vi "Color Editor.vi"(9 "Min":sgl, 10 "Max":sgl=10.0, 11 "Color Ramp Cluster in":T1={"Color Ramp Style"=enum."None", "Color Ramp Array"=[16711934, 393471, 57855, 4390754, 16449346, 16744722, 16711680], "Color Ramp Index"=[45, 91, 133, 175, 219, 255], "Interpolate?"=FALSE, "Logarithm?"=FALSE}) -> (3 "Color Ramp Cluster out":T1={"Color Ramp Style"=enum."None", "Color Ramp Array"=[16711934, 393471, 57855, 4390754, 16449346, 16744722, 16711680], "Color Ramp Index"=[45, 91, 133, 175, 219, 255], "Interpolate?"=FALSE, "Logarithm?"=FALSE})   [LabVIEW 2020, in "3D Plot.lvclass"]
uses:
  <vilib>/Math Plots/3D Math Plots/3D Plot/3D Plot/3D Plot.lvclass
  <vilib>/Math Plots/3D Math Plots/3D Plot/3D Plot/Typedef/Color Ramp Cluster.ctl
  <vilib>/Math Plots/3D Math Plots/3D Plot/3D Plot/Typedef/Color Editor State.ctl
panel:
  in  "Tab Control":enum32{"UI", "Input & Output"}(tab)
  in  "Help":bool
  out "Intensity Graph":dbl[][](graph)
  in  "Slider 10":i32(slide) scale=0.0..255.0
  in  "Numeric 10":sgl=50.0
  in  "Color 10":u32(colorbox)=6618880
  in  "Slider 9":i32(slide) scale=0.0..255.0
  in  "Numeric 9":sgl=50.0
  in  "Color 9":u32(colorbox)=6618880
  in  "Slider 8":i32(slide) scale=0.0..255.0
  in  "Numeric 8":sgl=50.0
  in  "Color 8":u32(colorbox)=6618880
  in  "Slider 7":i32(slide) scale=0.0..255.0
  in  "Numeric 7":sgl=50.0
  in  "Color 7":u32(colorbox)=6618880
  in  "Slider 6":i32(slide) scale=0.0..255.0
  in  "Numeric 6":sgl=50.0
  in  "Color 6":u32(colorbox)=6618880
  in  "Slider 5":i32(slide) scale=0.0..255.0
  in  "Numeric 5":sgl=50.0
  in  "Color 5":u32(colorbox)=6618880
  in  "Slider 4":i32(slide) scale=0.0..255.0
  in  "Numeric 4":sgl=50.0
  in  "Color 4":u32(colorbox)=6618880
  in  "Slider 3":i32(slide) scale=0.0..255.0
  in  "Numeric 3":sgl=50.0
  in  "Color 3":u32(colorbox)=6618880
  in  "Slider 2":i32(slide) scale=0.0..255.0
  in  "Numeric 2":sgl=50.0
  in  "Color 2":u32(colorbox)=6618880
  in  "Slider 1":i32(slide) scale=0.0..255.0
  in  "Numeric 1":sgl=50.0
  in  "Color 1":u32(colorbox)=6618880
  in  "Logarithm":bool
  in  "Interpolate":bool
  in  "Bottom Numeric":sgl
  in  "Top Numeric":sgl=100.0
  in  "Bottom Color":u32(colorbox)=16860
  in  "Top Color":u32(colorbox)=16711680
  in  "Delete":bool
  in  "Add":bool
  in  "Cancel":bool
  in  "OK":bool
  in  "Bounds Slider":cluster{u8, u8}(slide)={0, 255} scale=0.0..255.0
  in  "Active Slider ID":i32
  # "Color Ramp"
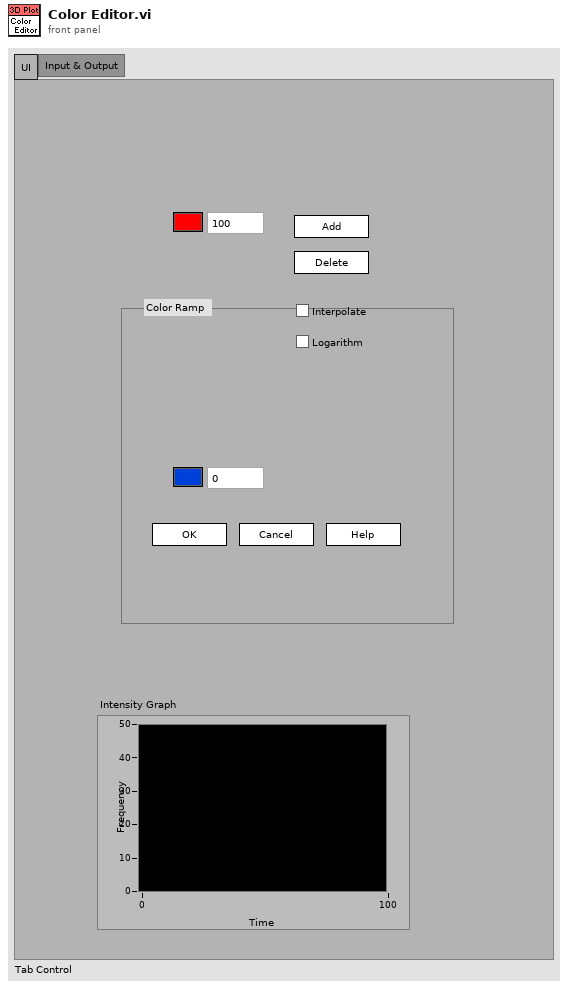
[diagram p1: front panel]
types:
  T1 = typedef "3D Plot.lvclass/Color Ramp Cluster.ctl" = cluster{"Color Ramp Style":enum16{"None", "Shaded", "Color spectrum", "Grey scale", "Custom"}, "Color Ramp Array":u32[], "Color Ramp Index":i32[], "Interpolate?":bool, "Logarithm?":bool}
  T2 = enum16{"None", "Shaded", "Color spectrum", "Grey scale", "Custom"}
  T3 = typedef "3D Plot.lvclass/Color Editor State.ctl" = enum16{"OK Pressed", "Cancel Pressed", "Update Color Ramp", "Update Height bySlider", "Update Height by Numeric", "Logarithm Color Ramp", "Set Active Slider", "Add a New Item", "Delete the Item"}
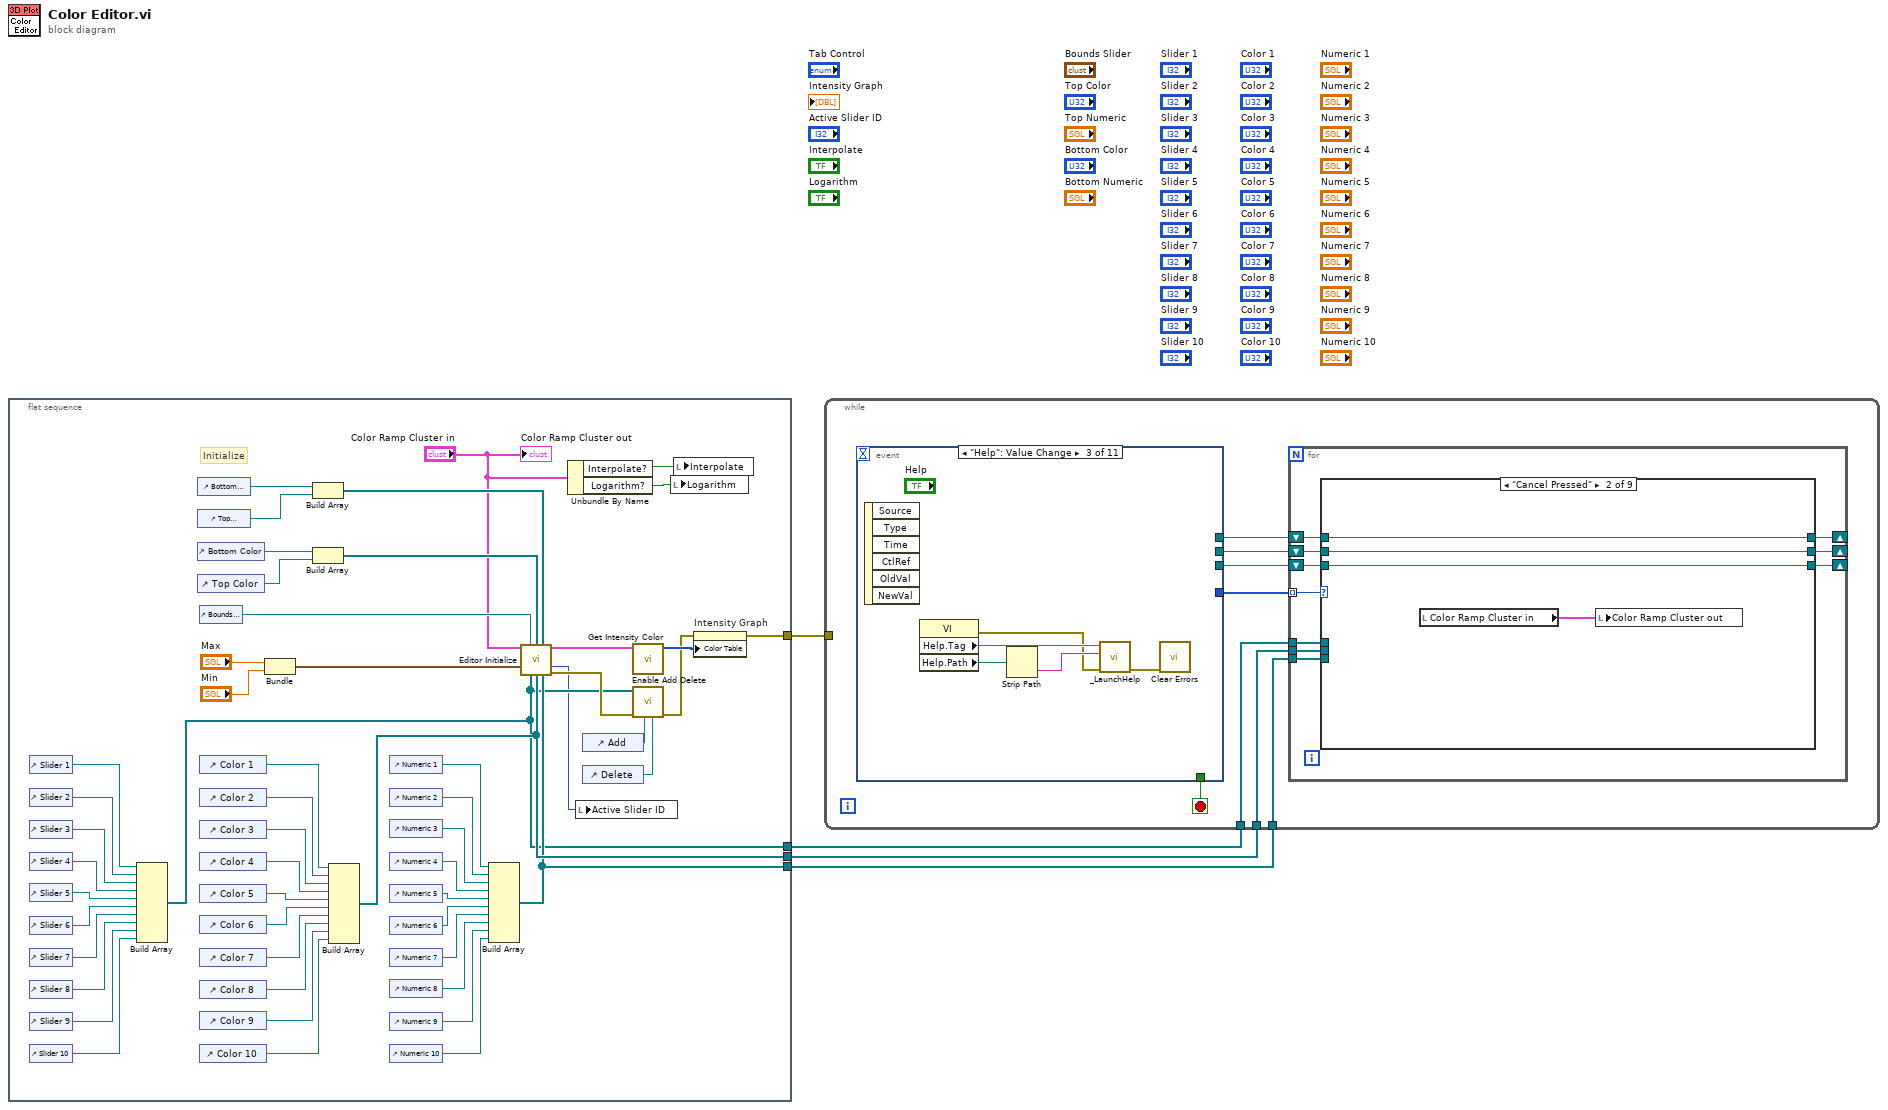
[diagram p0: block diagram]
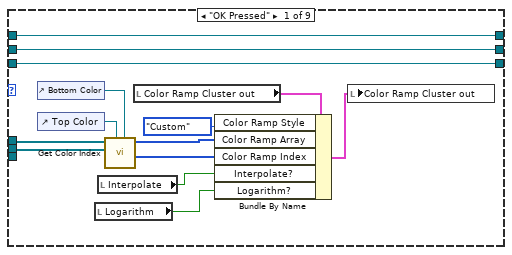
[diagram p2: hidden frame]
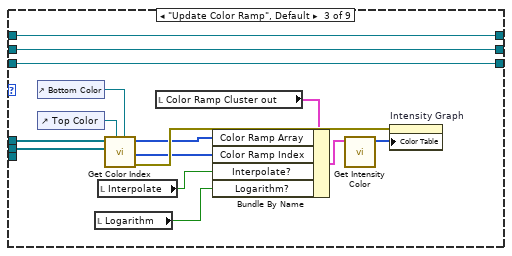
[diagram p3: hidden frame]
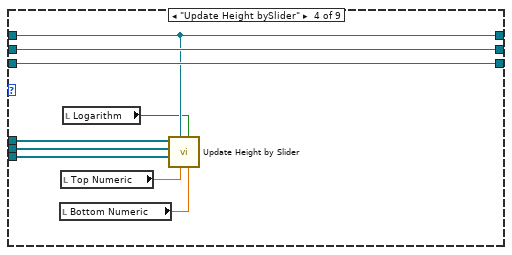
[diagram p4: hidden frame]
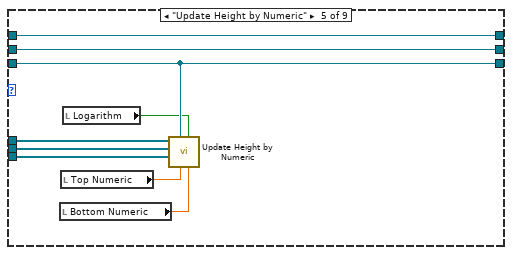
[diagram p5: hidden frame]
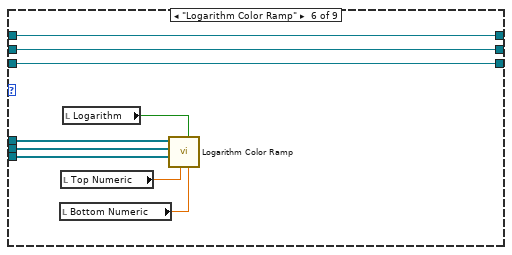
[diagram p6: hidden frame]
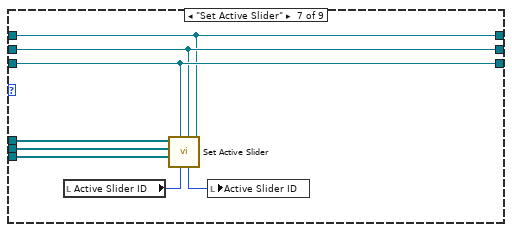
[diagram p7: hidden frame]
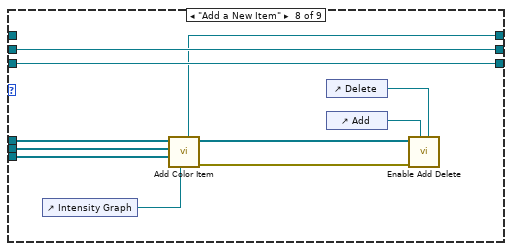
[diagram p8: hidden frame]
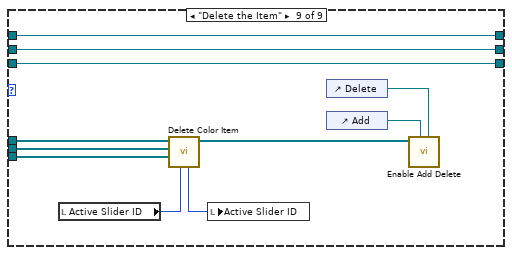
[diagram p9: hidden frame]
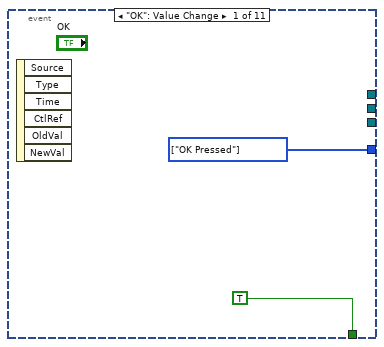
[diagram p10: hidden frame]
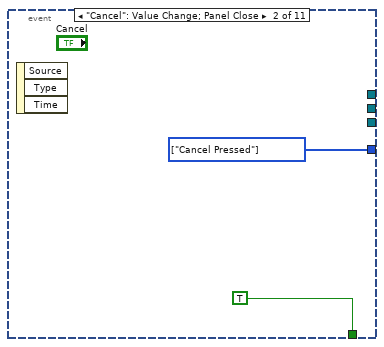
[diagram p11: hidden frame]
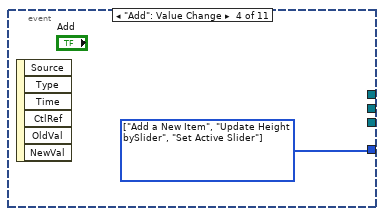
[diagram p12: hidden frame]
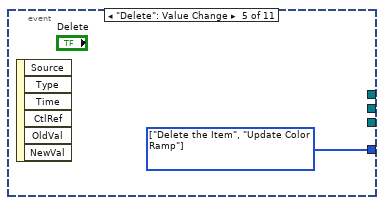
[diagram p13: hidden frame]
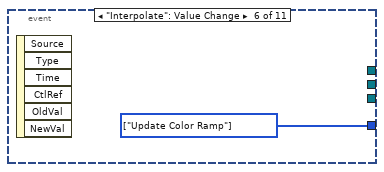
[diagram p14: hidden frame]
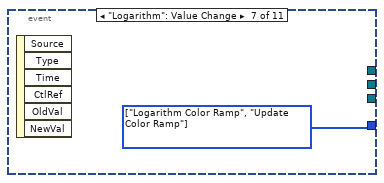
[diagram p15: hidden frame]
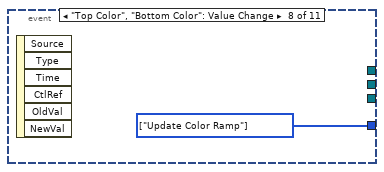
[diagram p16: hidden frame]
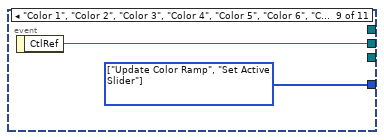
[diagram p17: hidden frame]
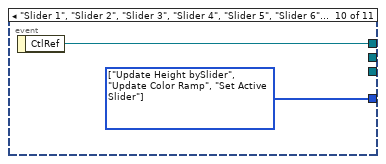
[diagram p18: hidden frame]
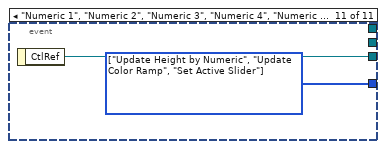
[diagram p19: hidden frame]
diagram:
  n1 = flat-sequence {
    tunnel: [w57] -> w4
    tunnel: [w10] -> w3
    tunnel: [w12] -> w2
    tunnel: [w11] -> w1
    frame #0 {
      # "Initialize"
      n2 = control-ref of="Slider 1"() -> (w21:refnum<vi>)
      n3 = control-ref of="Slider 2"() -> (w28:refnum<vi>)
      n4 = control-ref of="Slider 3"() -> (w29:refnum<vi>)
      n5 = control-ref of="Slider 4"() -> (w30:refnum<vi>)
      n6 = control-ref of="Slider 5"() -> (w31:refnum<vi>)
      n7 = control-ref of="Slider 6"() -> (w32:refnum<vi>)
      n8 = control-ref of="Slider 7"() -> (w33:refnum<vi>)
      n9 = control-ref of="Slider 8"() -> (w34:refnum<vi>)
      n10 = control-ref of="Slider 9"() -> (w35:refnum<vi>)
      n11 = control-ref of="Slider 10"() -> (w36:refnum<vi>)
      n12 = Build Array(w21, w28, w29, w30, w31, w32, w33, w34, w35, w36) -> (w10:refnum<vi>[])
      n13 = control-ref of="Bottom Numeric"() -> (w25:refnum<vi>)
      n14 = control-ref of="Top Numeric"() -> (w24:refnum<vi>)
      n15 = control-ref of="Bottom Color"() -> (w27:refnum<vi>)
      n16 = control-ref of="Top Color"() -> (w26:refnum<vi>)
      n17 = control-ref of="Bounds Slider"() -> (w20:refnum<vi>)
      n18 = control-ref of="Color 1"() -> (w47:refnum<vi>)
      n19 = control-ref of="Color 2"() -> (w48:refnum<vi>)
      n20 = control-ref of="Color 3"() -> (w49:refnum<vi>)
      n21 = control-ref of="Color 4"() -> (w50:refnum<vi>)
      n22 = control-ref of="Color 5"() -> (w51:refnum<vi>)
      n23 = control-ref of="Color 6"() -> (w52:refnum<vi>)
      n24 = control-ref of="Color 7"() -> (w53:refnum<vi>)
      n25 = control-ref of="Color 8"() -> (w54:refnum<vi>)
      n26 = control-ref of="Color 9"() -> (w55:refnum<vi>)
      n27 = control-ref of="Color 10"() -> (w56:refnum<vi>)
      n28 = Bundle("Max"="Max", "Min"="Min") -> (w15:cluster{"Max":sgl, "Min":sgl})  [unwired: 1 out]
      n29 = Build Array(w25, w24) -> (w22:refnum<vi>[])
      n30 = Build Array(w27, w26) -> (w23:refnum<vi>[])
      n31 = Build Array(w47, w48, w49, w50, w51, w52, w53, w54, w55, w56) -> (w12:refnum<vi>[])
      n32 = control-ref of="Numeric 1"() -> (w37:refnum<vi>)
      n33 = control-ref of="Numeric 2"() -> (w38:refnum<vi>)
      n34 = control-ref of="Numeric 3"() -> (w39:refnum<vi>)
      n35 = control-ref of="Numeric 4"() -> (w40:refnum<vi>)
      n36 = control-ref of="Numeric 5"() -> (w41:refnum<vi>)
      n37 = control-ref of="Numeric 6"() -> (w42:refnum<vi>)
      n38 = control-ref of="Numeric 7"() -> (w43:refnum<vi>)
      n39 = control-ref of="Numeric 8"() -> (w44:refnum<vi>)
      n40 = control-ref of="Numeric 9"() -> (w45:refnum<vi>)
      n41 = control-ref of="Numeric 10"() -> (w46:refnum<vi>)
      n42 = Build Array(w37, w38, w39, w40, w41, w42, w43, w44, w45, w46) -> (w11:refnum<vi>[])
      n43 = call <vilib>:"Editor Initialize.vi"("Color Ramp Cluster in"="Color Ramp Cluster in", "Fixed Slider Ref"=w20, "Fixed Color Ref Array"=w23, "Fixed Numeric Ref Array"=w22, "Range In"=w15, "Slider Ref Array"=w10, "Color Ref Array"=w12, "Numeric Ref Array"=w11) -> ("Color Ramp Cluster out"=w8:T1, "Active Slider ID"=w9:i32, "error out"=w14:errorcluster)  [unwired: 4 in, 1 out]
      n44 = Unbundle By Name("Color Ramp Cluster in") -> ("Interpolate?"=w7:bool, "Logarithm?"=w6:bool)
      n45 = local write "Active Slider ID"(w9) -> ()
      n46 = control-ref of="Add"() -> (w19:refnum<vi>)
      n47 = control-ref of="Delete"() -> (w18:refnum<vi>)
      n48 = call <vilib>:"Get Intensity Color.vi"("Color Ramp Cluster"=w8) -> ("Intensity Color"=w58:u32[])  [unwired: 4 in, 6 out]
      n49 = call <vilib>:"Enable Add Delete.vi"("Delete Ref"=w18, "Add Ref"=w19, "error in (no error)"=w14, "Slider Ref Array"=w10) -> ("error out"=w13:errorcluster)  [unwired: 7 out]
      n50 = local write "Logarithm"(w6) -> ()
      n51 = local write "Interpolate"(w7) -> ()
      n52 = property on="Intensity Graph" class="IntGraph (strict)"(error in=w13, "Color Table"=w58) -> (error out=w57:errorcluster)  [unwired: 1 in, 1 out]
      "Color Ramp Cluster out" <- "Color Ramp Cluster in"
    }
  }
  n53 = while {
    tunnel: w4 -> [_]
    tunnel: w1 -> [w62]
    tunnel: w2 -> [w65]
    tunnel: w3 -> [w63]
    stop <- w66 stop-if-true
    n54 = event shown="[2] \"Help\": Value Change" {
      selector: _ -> [_ _ _ _ _ _ _ _ _ _ _]
      dyn-events: _ -> [_ _ _ _ _ _ _ _ _ _ _]
      timeout: _ -> [_ _ _ _ _ _ _ _ _ _ _]
      tunnel: [TRUE TRUE ("OK") _ _ _ _ _ _ _ _ _] -> w66
      tunnel: [w166 w168 _ w174 w175 w176 w177 w178 w180 w181 w183] -> w64
      tunnel: [_ _ _ _ _ _ _ _ _ w182 _] -> w59
      tunnel: [_ _ _ _ _ _ _ _ _ _ w184] -> w60
      tunnel: [_ _ _ _ _ _ _ _ w179 _ _] -> w61
      event "OK": Value Change {
        w166 = T3[] [enum."OK Pressed"] items=["OK Pressed", "Cancel Pressed", "Update Color Ramp", "Update Height bySlider", "Update Height by Numeric", "Logarithm Color Ramp", "Set Active Slider", "Add a New Item", "Delete the Item"]
        n55 = event-data() -> ()  [unwired: 7 out]
      }
      event "Cancel": Value Change; Panel Close {
        w168 = T3[] [enum."Cancel Pressed"] items=["OK Pressed", "Cancel Pressed", "Update Color Ramp", "Update Height bySlider", "Update Height by Numeric", "Logarithm Color Ramp", "Set Active Slider", "Add a New Item", "Delete the Item"]
        n56 = event-data() -> ()  [unwired: 4 out]
      }
      event "Help": Value Change {
        n57 = event-data() -> ()  [unwired: 7 out]
        n58 = property class="VI"() -> (error out=w170:errorcluster, "Help.Tag"=w172:string, "Help.Path"=w173:path)  [unwired: 2 in, 1 out]
        n59 = Strip Path(path=w173) -> (name=w171:string)  [unwired: 1 out]
        n60 = call <helpdir>:"_LaunchHelp.vi"("error in (no error)"=w170, "CHM or HLP filename (lvdialog.chm)"=w171, "HTML filename"=w172) -> ("error out"=w169:errorcluster)  [unwired: 4 out]
        n61 = call <vilib>:"Clear Errors.vi"("error in (no error)"=w169) -> ()  [unwired: 5 in, 2 out]
      }
      event "Add": Value Change {
        w174 = T3[] [enum."Add a New Item", enum."Update Height bySlider", enum."Set Active Slider"] items=["OK Pressed", "Cancel Pressed", "Update Color Ramp", "Update Height bySlider", "Update Height by Numeric", "Logarithm Color Ramp", "Set Active Slider", "Add a New Item", "Delete the Item"]
        n62 = event-data() -> ()  [unwired: 7 out]
      }
      event "Delete": Value Change {
        w175 = T3[] [enum."Delete the Item", enum."Update Color Ramp"] items=["OK Pressed", "Cancel Pressed", "Update Color Ramp", "Update Height bySlider", "Update Height by Numeric", "Logarithm Color Ramp", "Set Active Slider", "Add a New Item", "Delete the Item"] ("Array")
        n63 = event-data() -> ()  [unwired: 7 out]
      }
      event "Interpolate": Value Change {
        w176 = T3[] [enum."Update Color Ramp"] items=["OK Pressed", "Cancel Pressed", "Update Color Ramp", "Update Height bySlider", "Update Height by Numeric", "Logarithm Color Ramp", "Set Active Slider", "Add a New Item", "Delete the Item"]
        n64 = event-data() -> ()  [unwired: 7 out]
      }
      event "Logarithm": Value Change {
        w177 = T3[] [enum."Logarithm Color Ramp", enum."Update Color Ramp"] items=["OK Pressed", "Cancel Pressed", "Update Color Ramp", "Update Height bySlider", "Update Height by Numeric", "Logarithm Color Ramp", "Set Active Slider", "Add a New Item", "Delete the Item"] ("Array")
        n65 = event-data() -> ()  [unwired: 7 out]
      }
      event "Top Color", "Bottom Color": Value Change {
        w178 = T3[] [enum."Update Color Ramp"] items=["OK Pressed", "Cancel Pressed", "Update Color Ramp", "Update Height bySlider", "Update Height by Numeric", "Logarithm Color Ramp", "Set Active Slider", "Add a New Item", "Delete the Item"]
        n66 = event-data() -> ()  [unwired: 7 out]
      }
      event "Color 1", "Color 2", "Color 3", "Color 4", "Color 5", "Color 6", "Color 7", "Color 8", "Color 9", "Color 10": Value Change {
        w180 = T3[] [enum."Update Color Ramp", enum."Set Active Slider"] items=["OK Pressed", "Cancel Pressed", "Update Color Ramp", "Update Height bySlider", "Update Height by Numeric", "Logarithm Color Ramp", "Set Active Slider", "Add a New Item", "Delete the Item"]
        n67 = event-data() -> ("CtlRef"=w179:refnum<vi>)  [unwired: 1 out]
      }
      event "Slider 1", "Slider 2", "Slider 3", "Slider 4", "Slider 5", "Slider 6", "Slider 7", "Slider 8", "Slider 9", "Slider 10": Value Change {
        w181 = T3[] [enum."Update Height bySlider", enum."Update Color Ramp", enum."Set Active Slider"] items=["OK Pressed", "Cancel Pressed", "Update Color Ramp", "Update Height bySlider", "Update Height by Numeric", "Logarithm Color Ramp", "Set Active Slider", "Add a New Item", "Delete the Item"]
        n68 = event-data() -> ("CtlRef"=w182:refnum<vi>)  [unwired: 1 out]
      }
      event "Numeric 1", "Numeric 2", "Numeric 3", "Numeric 4", "Numeric 5", "Numeric 6", "Numeric 7", "Numeric 8", "Numeric 9", "Numeric 10": Value Change {
        w183 = T3[] [enum."Update Height by Numeric", enum."Update Color Ramp", enum."Set Active Slider"] items=["OK Pressed", "Cancel Pressed", "Update Color Ramp", "Update Height bySlider", "Update Height by Numeric", "Logarithm Color Ramp", "Set Active Slider", "Add a New Item", "Delete the Item"]
        n69 = event-data() -> ("CtlRef"=w184:refnum<vi>)  [unwired: 1 out]
      }
    }
    n70 = for {
      tunnel: w63 -> [w76]
      tunnel: w65 -> [w75]
      tunnel: w64 -> [w74] mode=indexing
      tunnel: w62 -> [w73]
      shift-right: [w69] -> _
      shift-left: w59 -> [w70]
      shift-right: [w68] -> _
      shift-left: w61 -> [w72]
      shift-right: [w67] -> _
      shift-left: w60 -> [w71]
      n71 = case shown="\"Cancel Pressed\"" w74 {
        tunnel: w76 -> [w81 _ w107 w114 w125 w133 w144 w147 w157]
        tunnel: w75 -> [w80 _ w106 w116 w124 w132 w142 w153 w160]
        tunnel: w70 -> [w90 w93 w104 w111 w120 w136 w139 _ w164]
        tunnel: w73 -> [_ _ _ w115 w123 w131 w143 w152 w159]
        tunnel: w71 -> [w88 w91 w102 w112 w122 w134 w141 w150 w162]
        tunnel: w72 -> [w89 w92 w103 w113 w121 w135 w140 w151 w163]
        tunnel: [w90 w93 w104 w111 w120 w136 w139 w146 w164] -> w69
        tunnel: [w89 w92 w103 w113 w121 w135 w140 w151 w163] -> w68
        tunnel: [w88 w91 w102 w112 w122 w134 w141 w150 w162] -> w67
        frame "OK Pressed" {
          n72 = control-ref of="Bottom Color"() -> (w86:refnum<vi>)
          n73 = control-ref of="Top Color"() -> (w87:refnum<vi>)
          n74 = local read "Logarithm"() -> (w77:bool)
          n75 = local read "Interpolate"() -> (w78:bool)
          n76 = call <vilib>:"Get Color Index.vi"("Bottom Color Ref"=w86, "Top Color Ref"=w87, "Color Ref Array"=w80, "Slider Ref Array"=w81) -> ("Color Ramp Index"=w83:i32[], "Color Ramp Array"=w84:u32[])  [unwired: 1 in, 5 out]
          n77 = local read "Color Ramp Cluster out"() -> (w85:T1)
          n78 = Bundle By Name(cluster=w85, "Color Ramp Style"=T2."Custom", "Color Ramp Array"=w84, "Color Ramp Index"=w83, "Interpolate?"=w78, "Logarithm?"=w77) -> (w82:T1)
          n79 = local write "Color Ramp Cluster out"(w82) -> ()
        }
        frame "Cancel Pressed" {
          n80 = local read "Color Ramp Cluster in"() -> (w94:T1)
          n81 = local write "Color Ramp Cluster out"(w94) -> ()
        }
        frame "Update Color Ramp", Default {
          n82 = control-ref of="Bottom Color"() -> (w108:refnum<vi>)
          n83 = control-ref of="Top Color"() -> (w109:refnum<vi>)
          n84 = local read "Logarithm"() -> (w96:bool)
          n85 = local read "Interpolate"() -> (w97:bool)
          n86 = call <vilib>:"Get Color Index.vi"("Bottom Color Ref"=w108, "Top Color Ref"=w109, "Color Ref Array"=w106, "Slider Ref Array"=w107) -> ("error out"=w101:errorcluster, "Color Ramp Index"=w98:i32[], "Color Ramp Array"=w99:u32[])  [unwired: 1 in, 4 out]
          n87 = local read "Color Ramp Cluster out"() -> (w100:T1)
          n88 = Bundle By Name(cluster=w100, "Color Ramp Array"=w99, "Color Ramp Index"=w98, "Interpolate?"=w97, "Logarithm?"=w96) -> (w95:T1)
          n89 = call <vilib>:"Get Intensity Color.vi"("Color Ramp Cluster"=w95) -> ("Intensity Color"=w105:u32[])  [unwired: 4 in, 6 out]
          n90 = property on="Intensity Graph" class="IntGraph (strict)"(error in=w101, "Color Table"=w105) -> ()  [unwired: 1 in, 2 out]
        }
        frame "Update Height bySlider" {
          n91 = local read "Bottom Numeric"() -> (w118:sgl)
          n92 = local read "Top Numeric"() -> (w117:sgl)
          n93 = local read "Logarithm"() -> (w110:bool)
          n94 = call <vilib>:"Update Height by Slider.vi"("Bottom Numeric"=w118, "Logarithm?"=w110, "Top Numeric"=w117, "Slider Ref"=w111, "Numeric Ref Array"=w115, "Color Ref Array"=w116, "Slider Ref Array"=w114) -> ()  [unwired: 1 in, 4 out]
        }
        frame "Update Height by Numeric" {
          n95 = local read "Bottom Numeric"() -> (w127:sgl)
          n96 = local read "Top Numeric"() -> (w126:sgl)
          n97 = local read "Logarithm"() -> (w119:bool)
          n98 = call <vilib>:"Update Height by Numeric.vi"("Bottom Numeric"=w127, "Logarithm?"=w119, "Top Numeric"=w126, "Active Numeric Ref"=w122, "Numeric Ref Array"=w123, "Color Ref Array"=w124, "Slider Ref Array"=w125) -> ()  [unwired: 1 in, 4 out]
        }
        frame "Logarithm Color Ramp" {
          n99 = local read "Bottom Numeric"() -> (w128:sgl)
          n100 = local read "Top Numeric"() -> (w129:sgl)
          n101 = local read "Logarithm"() -> (w130:bool)
          n102 = call <vilib>:"Logarithm Color Ramp.vi"("Bottom Numeric"=w128, "Logarithm?"=w130, "Top Numeric"=w129, "Numeric Ref Array"=w131, "Color Ref Array"=w132, "Slider Ref Array"=w133) -> ()  [unwired: 1 in, 5 out]
        }
        frame "Set Active Slider" {
          n103 = local read "Active Slider ID"() -> (w138:i32)
          n104 = call <vilib>:"Set Active Slider.vi"("Slider Ref"=w139, "Color Ref"=w140, "Ex Active Slider ID"=w138, "Numeric Ref"=w141, "Numeric Ref Array"=w143, "Color Ref Array"=w142, "Slider Ref Array"=w144) -> ("New Active Slider ID"=w137:i32)  [unwired: 1 in, 3 out]
          n105 = local write "Active Slider ID"(w137) -> ()
        }
        frame "Add a New Item" {
          n106 = control-ref of="Intensity Graph"() -> (w154:refnum<vi>)
          n107 = call <vilib>:"Add Color Item.vi"("Color Ramp Ref"=w154, "Numeric Ref Array In"=w152, "Color Ref Array In"=w153, "Slider Ref Array"=w147) -> ("error out"=w145:errorcluster, "Slider Ref"=w146:refnum<vi>)  [unwired: 1 in, 5 out]
          n108 = control-ref of="Delete"() -> (w148:refnum<vi>)
          n109 = control-ref of="Add"() -> (w149:refnum<vi>)
          n110 = call <vilib>:"Enable Add Delete.vi"("Delete Ref"=w148, "Add Ref"=w149, "error in (no error)"=w145, "Slider Ref Array"=w147) -> ()  [unwired: 8 out]
        }
        frame "Delete the Item" {
          n111 = local read "Active Slider ID"() -> (w161:i32)
          n112 = call <vilib>:"Delete Color Item.vi"("Former Active Slider ID"=w161, "Numeric Ref Array In"=w159, "Color Ref Array In"=w160, "Slider Ref Array"=w157) -> ("New Active Slider ID"=w158:i32)  [unwired: 1 in, 6 out]
          n113 = local write "Active Slider ID"(w158) -> ()
          n114 = control-ref of="Delete"() -> (w155:refnum<vi>)
          n115 = control-ref of="Add"() -> (w156:refnum<vi>)
          n116 = call <vilib>:"Enable Add Delete.vi"("Delete Ref"=w155, "Add Ref"=w156, "Slider Ref Array"=w157) -> ()  [unwired: 1 in, 8 out]
        }
      }
    }
  }
